vi "HEWH Valve Start Setup.vi"(0 "MW100":refnum<visa-resource-name>, 2 "Valve Bank Setting":T4, 3 "Stop Intellifaucet?":bool, 4 "Pressurize Tank?":bool, 5 "error in (no error)":errorcluster, 7 "Debug":bool, 8 "Station ID":T2=enum."A", 9 "Refnum in":T1, 10 "LV Program":T3=enum."HEWH", 11 "Start Intellifaucet?":bool) -> (14 "dup VISA session":refnum<visa-resource-name>, 19 "error out":errorcluster)   [LabVIEW 2016]
uses:
  Type Definitions/HEWH Valve Bank Positions.ctl
  Utility/Save File/File Setup (Public)/Type Definition/Save File DOE LabView Program.ctl
  Custom Instrument Control/MW100/Type Definitions/Station ID Selector.ctl
  Type Definitions/HEWH Normally Open Valve Control.ctl
  Utility/Save File/File Setup.lvlib
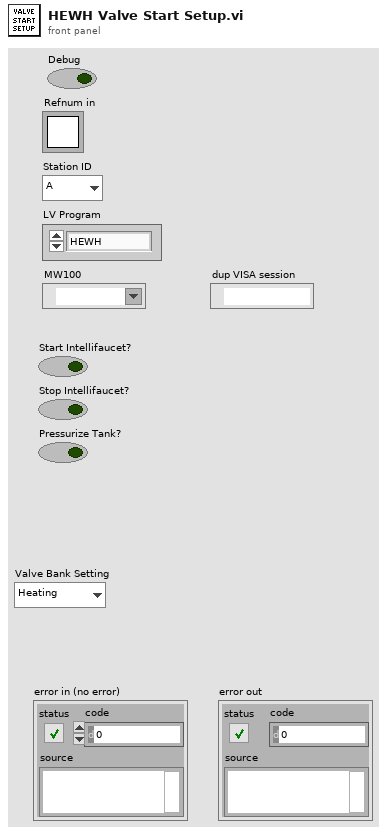
[diagram p1: front panel]
types:
  T1 = typedef "Semaphore RefNum" = refnum<k1>
  T2 = typedef "Station ID Selector.ctl" = enum16{"", "A", "B", "C", "D", "Global"}
  T3 = typedef "File Setup.lvlib/Save File DOE LabView Program.ctl" = enum16{"No Name Found", "DOE Stand", "Dishwasher Kitchen", "Portable Stand", "HEWH", "Dryer", "Dryer WILT", "HCC", "PRAT", "HEWH RLT", "Refrigeration"}
  T4 = typedef "HEWH Valve Bank Positions.ctl" = enum16{"Heating", "Purge", "Resting", "Draw"}
  T5 = typedef "HEWH Normally Open Valve Control.ctl" = string
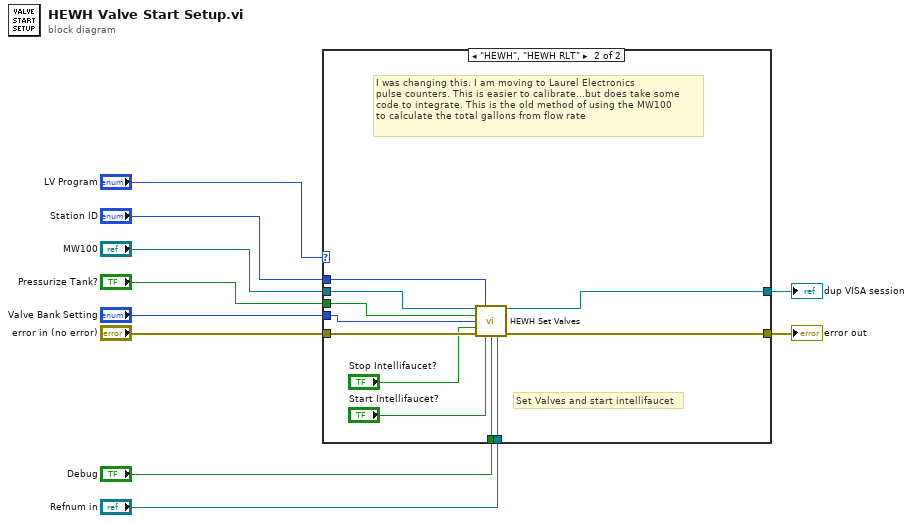
[diagram p0: block diagram]
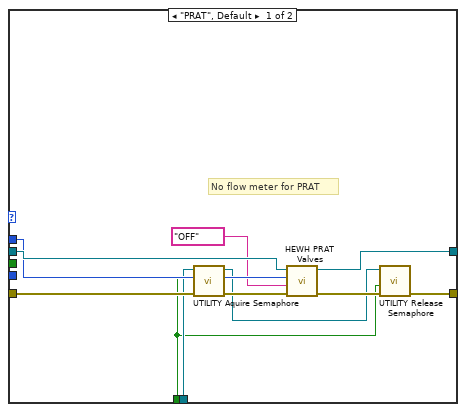
[diagram p2: hidden frame]
diagram:
  n1 = case shown="\"HEWH\", \"HEWH RLT\"" "LV Program" {
    tunnel: "Pressurize Tank?" -> [_ w32]
    tunnel: "Valve Bank Setting" -> [_ w31]
    tunnel: "error in (no error)" -> [w18 w30]
    tunnel: [w14 w22] -> w2
    tunnel: [w19 w23] -> w1
    tunnel: "MW100" -> [w21 w27]
    tunnel: "Station ID" -> [w20 w26]
    tunnel: "Debug" -> [w12 w25]
    tunnel: "Refnum in" -> [w16 w24]
    frame "PRAT", Default {
      # "No flow meter for PRAT"
      n2 = call "UTILITY Aquire Semaphore.vi"("error in (no error)"=w18, "Debug"=w12, "Refnum in"=w16) -> ("error out"=w17:errorcluster, "Refnum out"=w13:T1)  [unwired: 6 in, 1 out]
      n3 = call "HEWH PRAT Valves.vi"("error in (no error)"=w17, "Normally Open Valve"=T5 "OFF", "Station ID"=w20, "MW100 In"=w21) -> ("error out"=w15:errorcluster, "MW100 Out"=w19:refnum<visa-resource-name>)  [unwired: 6 in]
      n4 = call "UTILITY Release Semaphore.vi"("error in (no error)"=w15, "Debug"=w12, "Refnum in"=w13) -> ("error out"=w14:errorcluster)  [unwired: 8 in]
    }
    frame "HEWH", "HEWH RLT" {
      # "I was changing this. I am moving to Laurel Electronics\npulse counters. This is easier to calibrate...but does take some \ncode to integrate. This is the old method of using the MW100\nto calculate the total gallons from flow rate"
      # "Set Valves and start intellifaucet"
      n5 = call "HEWH Set Valves.vi"("VISA session"=w27, "Station ID"=w26, "Pressurize Tank?"=w32, "Valve Bank Setting"=w31, "Stop Intellifaucet?"="Stop Intellifaucet?", "Error In"=w30, "Start Intellifaucet?"="Start Intellifaucet?", "Debug"=w25, "Refnum in"=w24) -> ("dup VISA session"=w23:refnum<visa-resource-name>, "Error Out"=w22:errorcluster)  [unwired: 5 in]
    }
  }
  "error out" <- w2
  "dup VISA session" <- w1
